vi "Util_RetrieveNI-RT_ini.vi"(5 "password":string, 7 "user (admin)":string="admin", 8 "error in":errorcluster, 9 "Target settings":T1={"Hostname"="", "Serial number"="", "Product name"="", "Product code"=0, "System status"="", "Credential type"=enum."None/Unlocked", "User added?"=FALSE, "Primary NIC"={"MAC address"="", "IP Address Request Mode"=2, "IP address"="", "Subnet mask"="", "Gateway"="", "DNS server"=""}} {"Primary NIC"."IP Address Request Mode" items=["Static"=1, "DHCP/Link-Local"=2, "Link-Local Only"=4, "DHCP Only"=8]}, 11 "temp folder":path) -> (0 "error out":errorcluster, 3 "Ini File Path":path)   [LabVIEW 2016]
uses:
  Targets/TypeDefs/rad_Target Information.ctl
  Targets/TypeDefs/rad_Target Network Settings.ctl
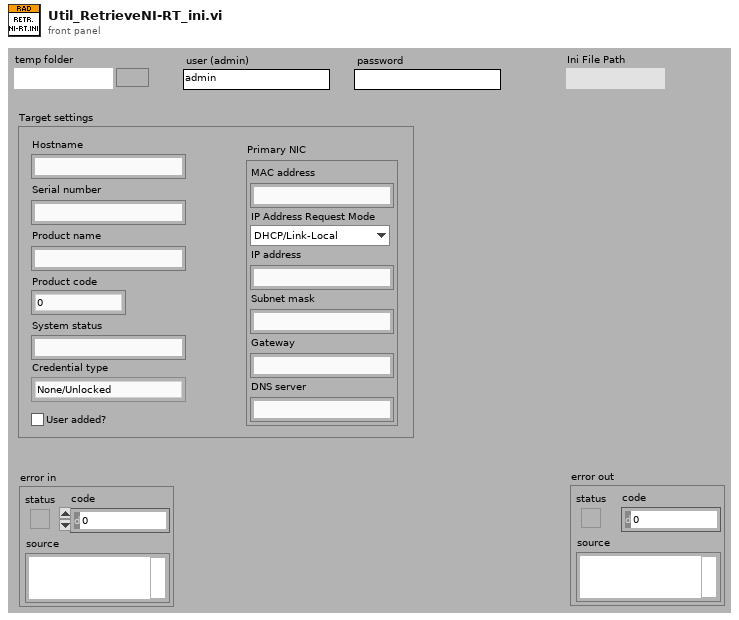
[diagram p1: front panel]
types:
  T1 = typedef "rad_Target Information.ctl" = cluster{"Hostname":string, "Serial number":string, "Product name":string, "Product code":i32, "System status":string, "Credential type":enum16{"None/Unlocked", "FTP Password", "NIAuth Credentials"}, "User added?":bool, "Primary NIC":T2}
  T2 = typedef "rad_Target Network Settings.ctl" = cluster{"MAC address":string, "IP Address Request Mode":i32, "IP address":string, "Subnet mask":string, "Gateway":string, "DNS server":string}
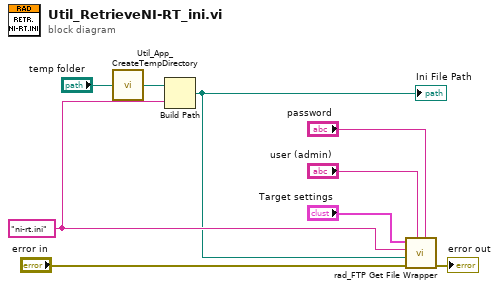
[diagram p0: block diagram]
diagram:
  w6 = "ni-rt.ini" ("Title")
  n1 = call "Util_App_CreateTempDirectory.vi"("TempFolderPath"="temp folder") -> ("TempFolderPath_out"=w5:path)
  n2 = Build Path(base path=w5, name or relative path=w6) -> (appended path=w2:path)
  "Ini File Path" <- w2
  n3 = call "rad_FTP Get File Wrapper.vi"("password"="password", "user (admin)"="user (admin)", "error in (no error)"="error in", "local path"=w2, "remote path"=w6, "Target settings"="Target settings") -> ("error out"=→"error out":errorcluster)  [unwired: 5 in]
